vi "Variable@CopyFromTo__Parameter.vi"(1 "ParamterIn":string) -> (0 "ParamterOut":string)   [LabVIEW 2020]
panel:
  in  "NewName":string(combo)
  in  "SectionTo":string(combo)
  in  "SectionFrom":string(combo)
  in  "ParameterName":string(combo)
  in  "Confirm":bool
  # "Variable@CopyFromTo $Variable,$Form,$To(,NewName)"
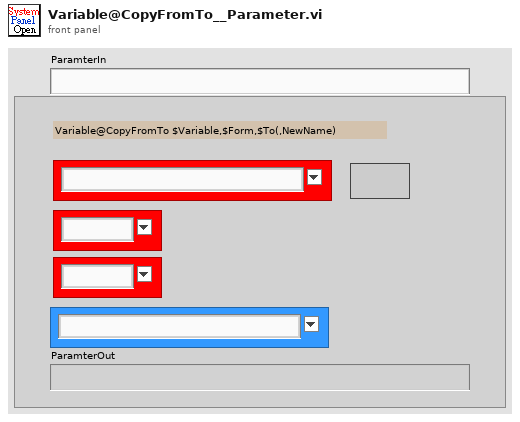
[diagram p1: front panel]
types:
  T1 = enum16{"Get", "Init", "Set", "Delete", "GetElement", "Inc", "Dec"}
  T2 = enum16{"Get", "Init", "Set", "Delete", "GetElement", "Inc", "Dec", "ReName"}
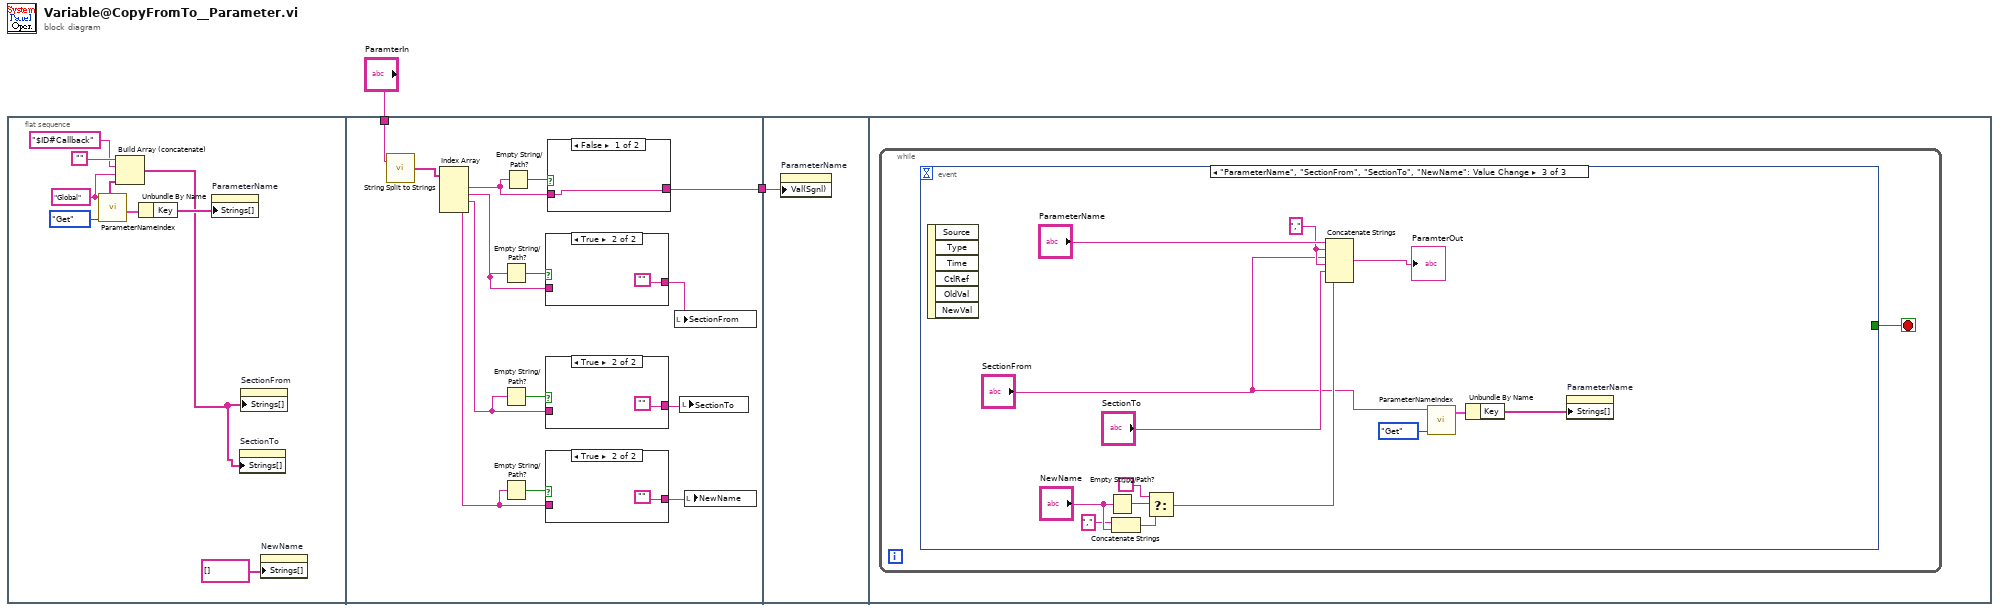
[diagram p0: block diagram]
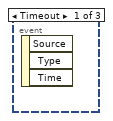
[diagram p6: hidden frame]
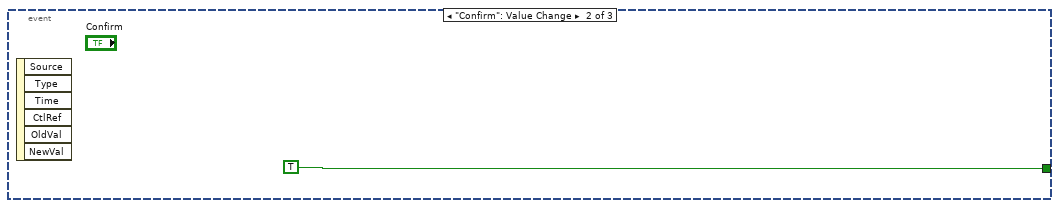
[diagram p7: hidden frame]
diagram:
  n1 = flat-sequence {
    tunnel: "ParamterIn" -> [w21]
    tunnel: [w23] -> w1
    tunnel: w1 -> [w34]
    frame #0 {
      w5 = "Global" ("VariableSection")
      n2 = call "ParameterNameIndex.vi"("OP"=T1."Get", "VariableSection"=w5) -> ("GlobalKeyValue"=w10:cluster{"Key":string[], "Value":string[]}, "SectionList"=w6:string[])  [unwired: 3 in, 5 out]
      n3 = Build Array (concatenate)("", "$ID#Callback" ("VariableSection"), w5, w6) -> (w4:string[])
      n4 = Unbundle By Name(w10) -> ("Key"=w9:string[])
      n5 = property on="ParameterName" class="CmbBox"("Strings[]"=w9) -> ()  [unwired: 2 in, 2 out]
      n6 = property on="SectionTo" class="CmbBox"("Strings[]"=w4) -> ()  [unwired: 2 in, 2 out]
      n7 = property on="SectionFrom" class="CmbBox"("Strings[]"=w4) -> ()  [unwired: 2 in, 2 out]
      n8 = property on="NewName" class="CmbBox"("Strings[]"=string[] [] ("Strings []")) -> ()  [unwired: 2 in, 2 out]
    }
    frame #1 {
      n9 = call "String Split to Strings.vi"("String"=w21) -> ("Array"=w20:string[])  [unwired: 1 in]
      n10 = Index Array(array=w20) -> (element #1=w19:string, element #2=w18:string, element #3=w16:string, element #4=w13:string)  [unwired: 4 in]
      n11 = Empty String/Path?(string/path=w18) -> (empty?=w24:bool)
      n12 = Empty String/Path?(string/path=w16) -> (empty?=w17:bool)
      n13 = Empty String/Path?(string/path=w13) -> (empty?=w14:bool)
      n14 = Empty String/Path?(string/path=w19) -> (empty?=w25:bool)
      n15 = case shown="True" w24 {
        tunnel: w18 -> [w30 _]
        tunnel: [w30 ""] -> w22
        frame False {
        }
        frame True {
        }
      }
      n16 = case shown="True" w17 {
        tunnel: w16 -> [w28 _]
        tunnel: [w28 ""] -> w15
        frame False {
        }
        frame True {
        }
      }
      n17 = case shown="True" w14 {
        tunnel: w13 -> [w26 _]
        tunnel: [w26 ""] -> w12
        frame False {
        }
        frame True {
        }
      }
      n18 = case shown="False" w25 {
        tunnel: w19 -> [w32 w33]
        tunnel: [w32 w33] -> w23
        frame False {
        }
        frame True {
        }
      }
      n19 = local write "SectionFrom"(w22) -> ()
      n20 = local write "SectionTo"(w15) -> ()
      n21 = local write "NewName"(w12) -> ()
    }
    frame #2 {
      n22 = property on="ParameterName" class="CmbBox"("Val(Sgnl)"=w34) -> ()  [unwired: 2 in, 2 out]
    }
    frame #3 {
      n23 = while {
        stop <- w35 stop-if-true
        n24 = event shown="[2] \"ParameterName\", \"SectionFrom\", \"SectionTo\", \"NewName\": Value Change" {
          selector: _ -> [_ _ _]
          dyn-events: _ -> [_ _ _]
          timeout: _ -> [_ _ _]
          tunnel: [_ TRUE _] -> w35
          event Timeout {
            n25 = event-data() -> ()  [unwired: 1 in, 3 out]
          }
          event "Confirm": Value Change {
            n26 = event-data() -> ()  [unwired: 1 in, 6 out]
          }
          event "ParameterName", "SectionFrom", "SectionTo", "NewName": Value Change {
            w48 = "," ("string")
            n27 = event-data() -> ()  [unwired: 1 in, 6 out]
            n28 = Empty String/Path?(string/path="NewName") -> (empty?=w45:bool)
            n29 = Concatenate Strings("," ("string"), "NewName") -> (w43:string)
            n30 = Select(t="", s=w45, f=w43) -> (s? t:f=w40:string)
            n31 = Concatenate Strings("ParameterName", w48, "SectionFrom", w48, "SectionTo", w40) -> (→"ParamterOut":string)
            n32 = call "ParameterNameIndex.vi"("OP"=T2."Get", "VariableSection"="SectionFrom") -> ("SectionKeyValue"=w38:cluster{"Key":string[], "Value":string[]})  [unwired: 3 in, 6 out]
            n33 = Unbundle By Name(w38) -> ("Key"=w46:string[])
            n34 = property on="ParameterName" class="CmbBox"("Strings[]"=w46) -> ()  [unwired: 2 in, 2 out]
          }
        }
      }
    }
  }
